vi "PH_Beckhoff_PP_Control.get PP Conductivity Tagname.vi"(1 "PP Conductivity Tag":T1) -> (0 "PP Conductivity Tagname":string)   [LabVIEW 2014, in "PH_Beckhoff_PP_Control.lvlib"]
doc: "This VI concatenates a Tagname out of strict type def enum controls. It keeps also the information whether the Tag is existing (if not, N/A is given out as name)."
uses:
  PH_Beckhoff_PP_Control.lvlib
  PH_Beckhoff_PP_Control.PP Conductivity Tags.ctl
  PH_Common/Names/PH_Names.Subsystems.ctl
  PH_PP_Common/PH_PP_Common.Devices.ctl
  PH_Common/Names/PH_Names.Communication Type.ctl
  PH_Common/PH_Common.lvlib
  PH_PP_Common/PH_PP_Common.lvlib
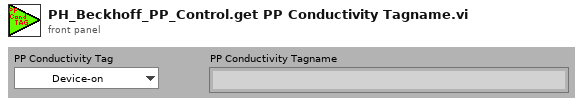
[diagram p1: front panel]
types:
  T1 = typedef "PH_Beckhoff_PP_Control.lvlib/PH_Beckhoff_PP_Control.PP Conductivity Tags.ctl" = enum16{"Device-on", "Conductivity-2-high", "Temperature-not-2-low", "Alarm", "Conductivity", "Status"}
  T2 = typedef "PH_PP_Common.lvlib/PH_PP_Common.Devices.ctl" = enum16{"no Info", "Igni", "RR", "DumpRoss", "PSU", "Trigger", "HV-Meas", "Rods", "Chiller", "Conductivity", "Mercury"}
  T3 = typedef "PH_Common.lvlib/PH_Names.Subsystems.ctl" = enum16{"no Info", "fs-FE", "ns-FE", "PA", "MA", "MAS", "COS", "Exp-LB", "Exp-LL", "PP", "PILS"}
  T4 = typedef "PH_Common.lvlib/PH_Names.Communication Type.ctl" = enum16{"no Info", "SE", "SA", "AE", "AA", "DE", "DA", "DIM"}
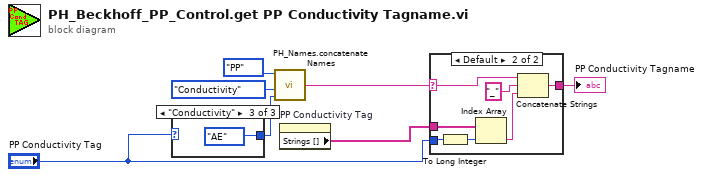
[diagram p0: block diagram]
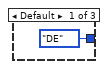
[diagram p2: hidden frame]
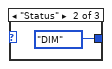
[diagram p3: hidden frame]
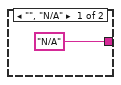
[diagram p4: hidden frame]
diagram:
  n1 = case shown="\"Conductivity\"" "PP Conductivity Tag" {
    tunnel: [PH_Names.Communication_Type."DE" ("Communication Type (no info)") PH_Names.Communication_Type."DIM" ("Communication Type (no info)") PH_Names.Communication_Type."AE" ("Communication Type (no info)")] -> w2
    frame Default {
    }
    frame "Status" {
    }
    frame "Conductivity" {
    }
  }
  n2 = call "PH_Names.concatenate Names.vi"("Communication Type (no info)"=w2, "Devices (no info)"=PH_PP_Common.Devices."Conductivity", "Subsystem"=PH_Names.Subsystems."PP") -> ("Subsystem_PU_Devices_Comm Type"=w6:string)  [unwired: 1 in]
  n3 = property on="PP Conductivity Tag" class="Enum (strict)"() -> ("Strings []"=w5:string[])  [unwired: 2 in, 2 out]
  n4 = case shown="Default" w6 {
    selector: w6 -> [_ w12]
    tunnel: ["N/A" w18] -> w7
    tunnel: w5 -> [_ w17]
    tunnel: "PP Conductivity Tag" -> [_ w13]
    frame "", "N/A" {
    }
    frame Default {
      n5 = To Long Integer(number=w13) -> (32bit integer=w16:i32)
      n6 = Index Array(array=w17, index=w16) -> (element=w15:string)
      n7 = Concatenate Strings(w12, "_" ("string"), w15) -> (w18:string)
    }
  }
  "PP Conductivity Tagname" <- w7
